vi "PLC Array Byte Stream to G Object 2.vi"(8 "error in (no error)":errorcluster, 9 "Array Type Descriptor":T1, 10 "Byte Stream":u8[](array[numeric]), 11 "TwinCAT ADS in":refnum<class "TwinCAT ADS.lvclass">) -> (0 "error out":errorcluster, 2 "Value":variant, 3 "TwinCAT ADS out":refnum<class "TwinCAT ADS.lvclass">)   [LabVIEW 2018]
uses:
  TwinCAT ADS.lvclass
  Controls/PLC Type.ctl
  Controls/PLC Sub-Item Type Descriptor.ctl
  Controls/PLC Array Type Descriptor.ctl
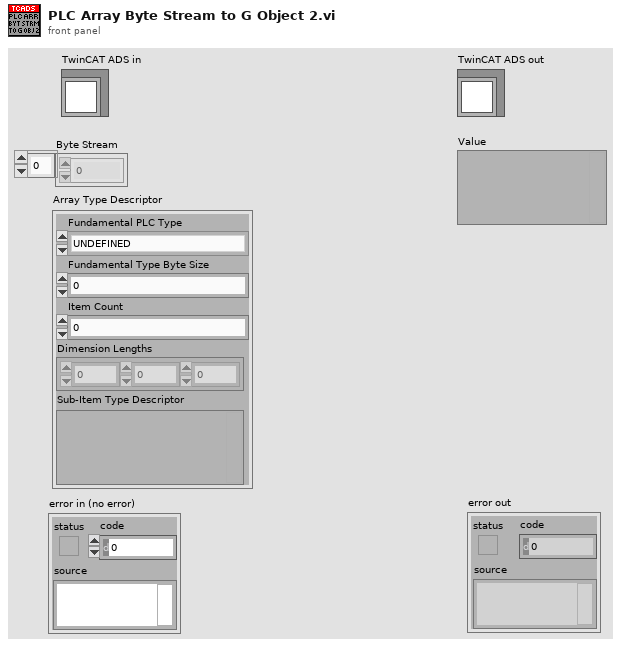
[diagram p1: front panel]
types:
  T1 = typedef "TwinCAT ADS.lvclass/PLC Array Type Descriptor.ctl" = cluster{"Fundamental PLC Type":T2, "Fundamental Type Byte Size":i32, "Item Count":i32, "Dimension Lengths":i32[], "Sub-Item Type Descriptor":variant}
  T2 = typedef "TwinCAT ADS.lvclass/PLC Type.ctl" = enum16{"UNDEFINED", "INT", "DINT", "REAL", "LREAL", "SINT", "BYTE", "UINT", "UDINT", "LINT", "ULINT", "STRING", "WSTRING", "BOOL", "TIME", "LTIME", "DATE", "DT", "TOD", "ARRAY", "JAGGED ARRAY", "STRUCT", "FUNCTION BLOCK", "POINTER", "USER DEFINED"}
  T3 = typedef "TwinCAT ADS.lvclass/PLC Sub-Item Type Descriptor.ctl" = cluster{"PLC Type":T2, "Offset":i32, "Byte Size":i32, "[Sub-Item/Array Type Descriptor]":variant[]}
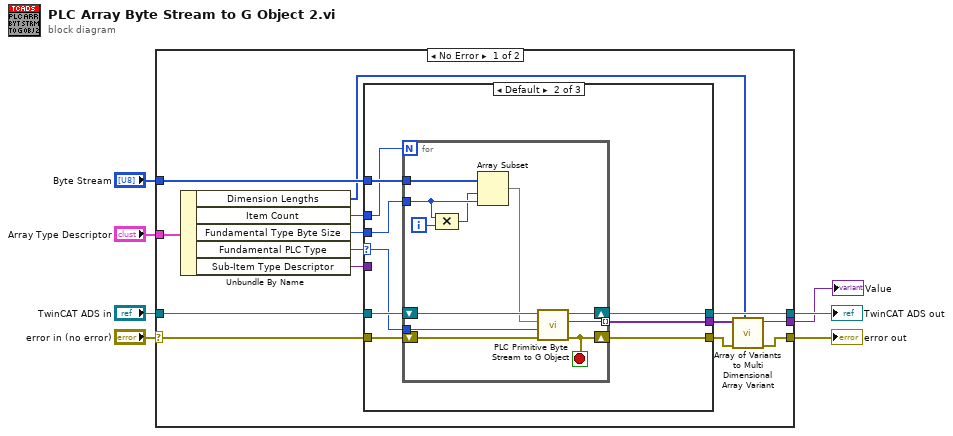
[diagram p0: block diagram]
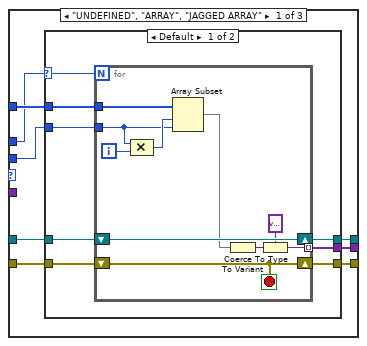
[diagram p2: hidden frame]
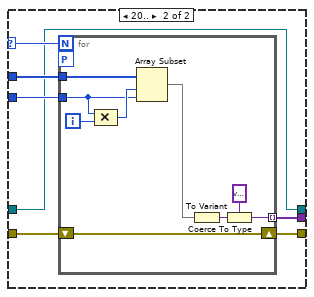
[diagram p3: hidden frame]
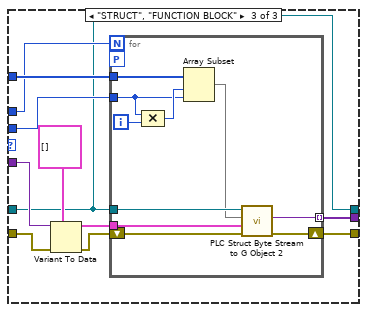
[diagram p4: hidden frame]
diagram:
  n1 = case shown="No Error" "error in (no error)" {
    selector: "error in (no error)" -> [w8 w105]
    tunnel: "TwinCAT ADS in" -> [w21 w106]
    tunnel: "Byte Stream" -> [w20 _]
    tunnel: [w18 w105] -> w5
    tunnel: [w17 w106] -> w4
    tunnel: [w16 _] -> w3
    tunnel: "Array Type Descriptor" -> [w14 _]
    frame No Error {
      n2 = Unbundle By Name(w14) -> ("Dimension Lengths"=w9:i32[], "Item Count"=w12:i32, "Fundamental Type Byte Size"=w10:i32, "Fundamental PLC Type"=w11:T2, "Sub-Item Type Descriptor"=w13:variant)
      n3 = case shown="Default" w11 {
        selector: w11 -> [_ w67 _]
        tunnel: w8 -> [w29 w72 w89]
        tunnel: w21 -> [w28 w71 w84]
        tunnel: w20 -> [w25 w65 w93]
        tunnel: [w26 w70 w94] -> w15
        tunnel: [w23 w69 w92] -> w19
        tunnel: [w27 w68 w84] -> w17
        tunnel: w13 -> [_ _ w88]
        tunnel: w12 -> [w22 w64 w91]
        tunnel: w10 -> [w24 w66 w90]
        frame "UNDEFINED", "ARRAY", "JAGGED ARRAY" {
          n4 = case shown="Default" w22 {
            selector: w22 -> [w30 w49]
            tunnel: w29 -> [w37 w54]
            tunnel: w28 -> [w36 w48]
            tunnel: [w35 w48] -> w27
            tunnel: [w34 w53] -> w26
            tunnel: w25 -> [w33 w52]
            tunnel: w24 -> [w32 w51]
            tunnel: [w31 w50] -> w23
            frame Default {
              n5 = for {
                N: w30 -> [_]
                shift-right: [w47] -> w35
                shift-left: w36 -> [w47]
                tunnel: w32 -> [w40]
                tunnel: [w44] -> w31 mode=indexing
                shift-right: [w46] -> w34
                shift-left: w37 -> [w46]
                tunnel: w33 -> [w42]
                i -> [w41]
                stop <- w46 stop-if-true
                n6 = Compound Arithmetic op=MULTIPLY(w40, w41) -> (w43:i32)
                n7 = Array Subset(array=w42, index=w43, length=w40) -> (w39:u8[])
                n8 = To Variant(anything=w39) -> (Variant=w38:variant)
                n9 = Coerce To Type(0:w38, 1:variant ("Value")) -> (2:w44:variant)
              }
            }
            frame 20.. {
              n10 = for {
                N: w49 -> [_]
                tunnel: w51 -> [w57]
                tunnel: [w61] -> w50 mode=indexing
                shift-right: [w63] -> w53
                shift-left: w54 -> [w63]
                tunnel: w52 -> [w59]
                workers-P: _ -> [_]
                i -> [w58]
                n11 = Compound Arithmetic op=MULTIPLY(w57, w58) -> (w60:i32)
                n12 = Array Subset(array=w59, index=w60, length=w57) -> (w56:u8[])
                n13 = To Variant(anything=w56) -> (Variant=w55:variant)
                n14 = Coerce To Type(0:w55, 1:variant ("Value")) -> (2:w61:variant)
              }
            }
          }
        }
        frame Default {
          n15 = for {
            N: w64 -> [_]
            shift-right: [w81] -> w68
            shift-left: w71 -> [w82]
            tunnel: [w80] -> w69 mode=indexing
            tunnel: w67 -> [w79]
            tunnel: w66 -> [w75]
            shift-right: [w78] -> w70
            shift-left: w72 -> [w83]
            tunnel: w65 -> [w77]
            i -> [w76]
            stop <- w78 stop-if-true
            n16 = Compound Arithmetic op=MULTIPLY(w75, w76) -> (w74:i32)
            n17 = Array Subset(array=w77, index=w74, length=w75) -> (w73:u8[])
            n18 = call "PLC Primitive Byte Stream to G Object.vi"("error in (no error)"=w83, "PLC Type"=w79, "Byte Stream"=w73, "TwinCAT ADS in"=w82) -> ("error out"=w78:errorcluster, "Value"=w80:variant, "TwinCAT ADS out"=w81:refnum<class "TwinCAT ADS.lvclass">)  [unwired: 5 in]
          }
        }
        frame "STRUCT", "FUNCTION BLOCK" {
          n19 = Variant To Data(error in=w89, type=T3[] [] ("[Sub-Item Type Information]"), Variant=w88) -> (data=w85:T3[], error out=w87:errorcluster)
          n20 = for {
            N: w91 -> [_]
            tunnel: [w97] -> w92 mode=indexing
            tunnel: w90 -> [w101]
            tunnel: w85 -> [w95]
            shift-right: [w98] -> w94
            shift-left: w87 -> [w99]
            tunnel: w93 -> [w103]
            workers-P: _ -> [_]
            tunnel: w84 -> [w100]
            i -> [w102]
            n21 = Compound Arithmetic op=MULTIPLY(w101, w102) -> (w104:i32)
            n22 = Array Subset(array=w103, index=w104, length=w101) -> (w96:u8[])
            n23 = call "PLC Struct Byte Stream to G Object 2.vi"("error in (no error)"=w99, "[Sub-Item Type Information]"=w95, "Byte Stream"=w96, "TwinCAT ADS in"=w100) -> ("error out"=w98:errorcluster, "Value"=w97:variant)  [unwired: 5 in, 1 out]
          }
        }
      }
      n24 = call "Array of Variants to Multi Dimensional Array Variant.vi"("Dimension Lengths"=w9, "error in (no error)"=w15, "[Variant]"=w19) -> ("error out"=w18:errorcluster, "Array Variant"=w16:variant)  [unwired: 7 in]
    }
    frame Error {
    }
  }
  "error out" <- w5
  "Value" <- w3
  "TwinCAT ADS out" <- w4
